vi "Items.vi"(11 "MsgPackMessage in":refnum<class "WampMessage MsgPack.lvclass">) -> (2 "Bytes":u8[](array[numeric]), 3 "MsgPackMessage out":refnum<class "WampMessage MsgPack.lvclass">)   [LabVIEW 2020, in "wamplv.lvlib" / "WampMessage MsgPack.lvclass"]
uses:
  WampMessage MsgPack.lvclass
  WampMessage MsgPack.lvclass/WampMessage MsgPack.ctl
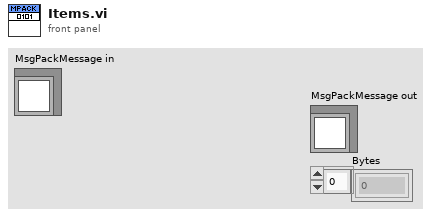
[diagram p1: front panel]
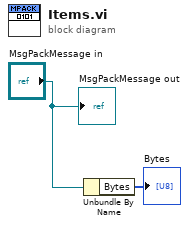
[diagram p0: block diagram]
diagram:
  n1 = Unbundle By Name("MsgPackMessage in") -> ("Bytes"=→"Bytes":u8[])
  "MsgPackMessage out" <- "MsgPackMessage in"
